vi "SubVI Nivel a Frecuencia.vi"(11 "UInt16":u16) -> (3 "Numeric":dbl)   [LabVIEW 2013]
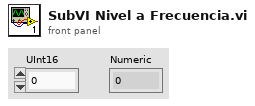
[diagram p1: front panel]
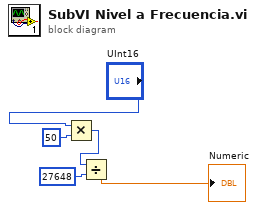
[diagram p0: block diagram]
diagram:
  n1 = Multiply(x="UInt16", y=50) -> (x*y=w3:i32)
  n2 = Divide(x=w3, y=27648) -> (x/y=→"Numeric":dbl)
